vi "Set Cluster Values from JSON String.vi"(8 "error in (no error)":errorcluster, 10 "JSON string":string="{\"TriggerActivation\":1,\n\"IRFormat\":2,\n\"TriggerSource\":3,\n\"TriggerSelector\":4,\n\"AcquisitionMode\":5,\n\"IncompleteBufferMode\":6,\n\"OutputImageType\":7,\n\"Timeout\":8,\n\"NUCMode\":9,\n\"NoiseReduction\":10,\n\"FocusPos\":11,\n\"AcquisitionFrameCount\":12,\n\"AcquisitionFrameRate\":10.0,\n\"TriggerMode\":13}", 11 "cluster reference":refnum<vi>) -> (0 "error out":errorcluster)   [LabVIEW 2023]
uses:
  <vilib>/Utility/Data Type/NI_Data Type.lvlib
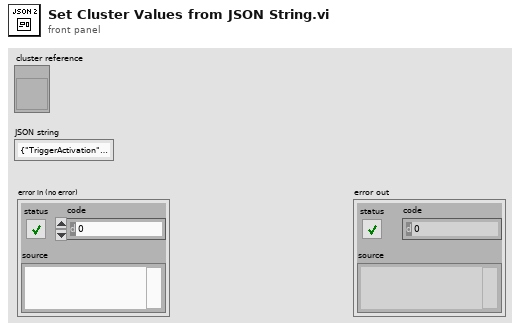
[diagram p1: front panel]
types:
  T1 = typedef "NI_Data Type.lvlib/Data Type.ctl" = enum8{"Invalid Type", "Void", "I8", "I16", "I32", "I64", "U8", "U16", "U32", "U64", "Single Float", "Double Float", "Extended Float", "Single Complex", "Double Complex", "Extended Complex", "Enum U8", "Enum U16", "Enum U32", "Enum U64", "Single Float With Unit", "Double Float With Unit", "Extended Float With Unit", "Single Complex with Unit", "Double Complex with Unit", "Extended Complex with Unit", "Boolean", "String", "Path", "Picture", "Tag", "Array", "Cluster", "Variant", "LV Variant", "Waveform", "Timestamp", "Digital Waveform", "Digital Data", "ExpressData", "Refnum", "External Data", "VI", "Poly VI", "LabVIEW Class Instance", "Fixed Point", "Set Collection", "Map Collection"}
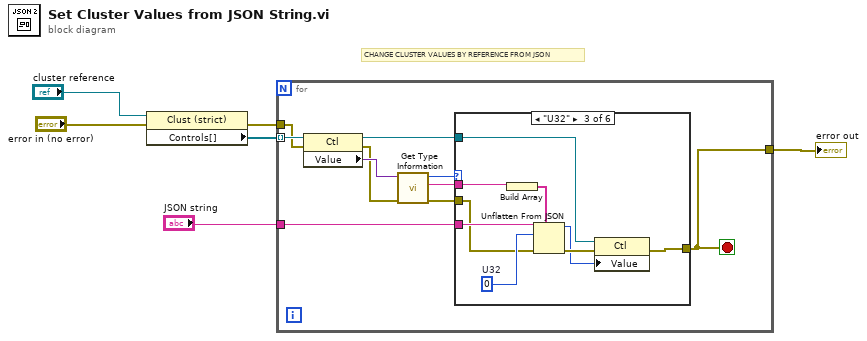
[diagram p0: block diagram]
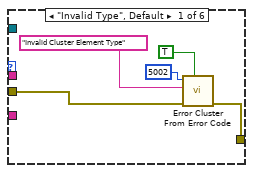
[diagram p2: hidden frame]
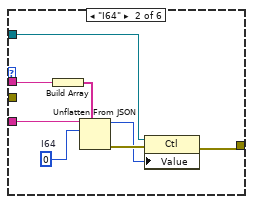
[diagram p3: hidden frame]
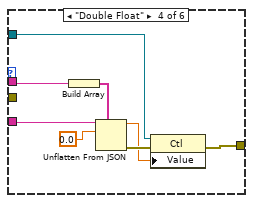
[diagram p4: hidden frame]
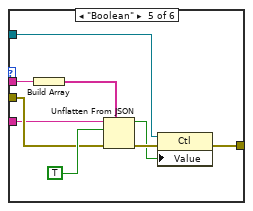
[diagram p5: hidden frame]
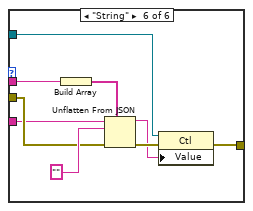
[diagram p6: hidden frame]
diagram:
  # "CHANGE CLUSTER VALUES BY REFERENCE FROM JSON"
  n1 = property class="Clust (strict)"(reference="cluster reference", error in="error in (no error)") -> (error out=w3:errorcluster, "Controls[]"=w5:refnum<vi>[])  [unwired: 1 out]
  n2 = for {
    tunnel: "JSON string" -> [w16]
    tunnel: w5 -> [w15] mode=indexing
    tunnel: w3 -> [w11]
    tunnel: [w7] -> w1
    stop <- w7 stop-if-true
    n3 = property class="Ctl"(reference=w15, error in=w11) -> (reference out=w8:refnum<vi>, error out=w10:errorcluster, "Value"=w14:variant)
    n4 = call <vilib>:"Get Type Information.vi"("error in (no error)"=w10, "variant"=w14) -> ("error out"=w9:errorcluster, "name"=w12:string, "type"=w13:T1)  [unwired: 5 in, 2 out]
    n5 = case shown="\"U32\"" w13 {
      tunnel: w16 -> [_ w27 w36 w44 w52 w59]
      tunnel: w12 -> [_ w26 w35 w43 w53 w58]
      tunnel: w9 -> [w18 _ w34 _ w54 w60]
      tunnel: w8 -> [_ w24 w30 w41 w49 w57]
      tunnel: [w21 w22 w31 w39 w47 w56] -> w7
      frame "Invalid Type", Default {
        n6 = call <vilib>:"Error Cluster From Error Code.vi"("show call chain? (False)"=TRUE, "error in (no error)"=w18, "error message (\"\")"="Invalid Cluster Element Type" ("error message (\"\")"), "error code (0)"=5002) -> ("error out"=w21:errorcluster)  [unwired: 5 in]
      }
      frame "I64" {
        w29 = i64 0  # I64
        n7 = Build Array(w26) -> (w28:string[])
        n8 = Unflatten From JSON(path=w28, JSON string=w27, type and defaults=w29) -> (value=w23:i64, error out=w25:errorcluster)  [unwired: 4 in]
        n9 = property class="Ctl"(reference=w24, error in=w25, "Value"=w23) -> (error out=w22:errorcluster)  [unwired: 1 out]
      }
      frame "U32" {
        w38 = u32 0  # U32
        n10 = Build Array(w35) -> (w37:string[])
        n11 = Unflatten From JSON(path=w37, JSON string=w36, type and defaults=w38, error in (no error)=w34) -> (value=w32:u32, error out=w33:errorcluster)  [unwired: 3 in]
        n12 = property class="Ctl"(reference=w30, error in=w33, "Value"=w32) -> (error out=w31:errorcluster)  [unwired: 1 out]
      }
      frame "Double Float" {
        n13 = Build Array(w43) -> (w45:string[])
        n14 = Unflatten From JSON(path=w45, JSON string=w44, type and defaults=0.0) -> (value=w40:dbl, error out=w42:errorcluster)  [unwired: 4 in]
        n15 = property class="Ctl"(reference=w41, error in=w42, "Value"=w40) -> (error out=w39:errorcluster)  [unwired: 1 out]
      }
      frame "Boolean" {
        n16 = Build Array(w53) -> (w51:string[])
        n17 = Unflatten From JSON(path=w51, JSON string=w52, type and defaults=TRUE, error in (no error)=w54) -> (value=w48:bool, error out=w50:errorcluster)  [unwired: 3 in]
        n18 = property class="Ctl"(reference=w49, error in=w50, "Value"=w48) -> (error out=w47:errorcluster)  [unwired: 1 out]
      }
      frame "String" {
        n19 = Build Array(w58) -> (w63:string[])
        n20 = Unflatten From JSON(path=w63, JSON string=w59, type and defaults="", error in (no error)=w60) -> (value=w61:string, error out=w62:errorcluster)  [unwired: 3 in]
        n21 = property class="Ctl"(reference=w57, error in=w62, "Value"=w61) -> (error out=w56:errorcluster)  [unwired: 1 out]
      }
    }
  }
  "error out" <- w1
